vi "GRNF_Joystick.vi"(7 "RefNum Name":string="My Motor RefNum") -> (0 "Error":errorcluster, 3 "Device Reference":T1)   [LabVIEW 2019]
uses:
  <vilib>/Rock Robotics/WPI/Joystick/WPI_JoystickDevRef.ctl
  <vilib>/Rock Robotics/WPI/Joystick/WPI_JoystickDeviceEnum.ctl
  <vilib>/Rock Robotics/WPI/Utilities/WPI_GetSetVariantRefNum.vi
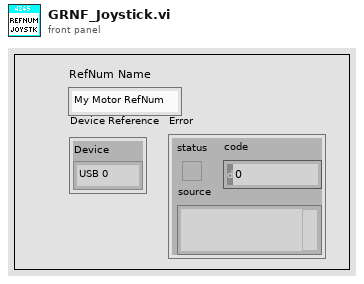
[diagram p1: front panel]
types:
  T1 = typedef "WPI_JoystickDevRef.ctl" = cluster{"Device":T2}
  T2 = typedef "WPI_JoystickDeviceEnum.ctl" = enum16{"USB 0", "USB 1", "USB 2", "USB 3", "USB 4", "USB 5"}
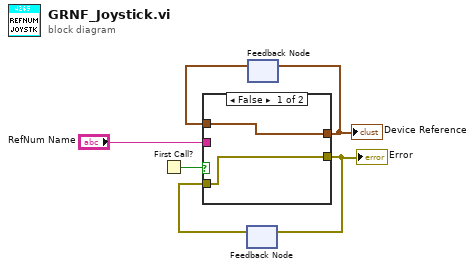
[diagram p0: block diagram]
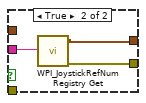
[diagram p2: hidden frame]
diagram:
  n1 = First Call?() -> (First Call?: T/F=w6:bool)
  n2 = feedback #1() -> (w1:errorcluster)  [unwired: 1 in]
  n3 = feedback #2() -> (w5:T1)  [unwired: 1 in]
  n4 = case shown="False" w6 {
    tunnel: [w8 w10] -> w4
    tunnel: w5 -> [w8 _]
    tunnel: "RefNum Name" -> [_ w11]
    tunnel: [w7 w9] -> w2
    tunnel: w1 -> [w7 _]
    frame False {
    }
    frame True {
      n5 = call <vilib>:"WPI_JoystickRefNum Registry Get.vi"("refnum name"=w11) -> ("error out"=w9:errorcluster, "JoystickDevRef"=w10:T1)  [unwired: 9 in]
    }
  }
  "Device Reference" <- w4
  "Error" <- w2
  n6 = feedback-in #1(w2) -> ()
  n7 = feedback-in #2(w4) -> ()
